vi "launcher.vi"(5 "RPM Control":dbl(knob) scale=0.0..3600.0, 6 "Stall":bool, 7 "Period (sec)":dbl) -> (0 "RPM":dbl(knob) scale=0.0..3000.0, 1 "RPM Steady?":bool, 3 "Motor Output":dbl(slide) scale=0.0..1.0)   [LabVIEW 2011]
uses:
  Robot Global Data.vi
  <vilib>/addons/control/pid/pid.llb/PID (DBL).vi
  <vilib>/addons/control/pid/NI_PID_pid.lvlib
panel:
  out "RPM Tolerance":dbl=25.0
  in  "PID Floor":dbl(knob)=609.2841617797657 scale=0.0..1000.0
  out "RPM High":bool
  out "RPM Low":bool
  out "1 RPM":bool
  out "5 RPM":bool
  out "2 RPM":bool
  out "8 RPM":bool
  out "7 RPM":bool
  out "6 RPM":bool
  out "4 RPM":bool
  out "3 RPM":bool
  out "RPM Control Response":cluster{"RPM Control 2":dbl, dbl, dbl}(graph)
  in  "Prop (like D)":dbl(knob)=0.002835162167809198 scale=0.0..0.01
  in  "Int (like P)":dbl(knob)=0.013165882226819458 scale=0.0..0.2
  in  "Deriv (not used)":dbl(knob) scale=0.0..0.01
  out "PID Output":dbl(graph)
  # "CIM: P=0.00192, I=0.00933, D=0.0"
  # "BB775: P=0.00283, I=0.01312, D=0.0"
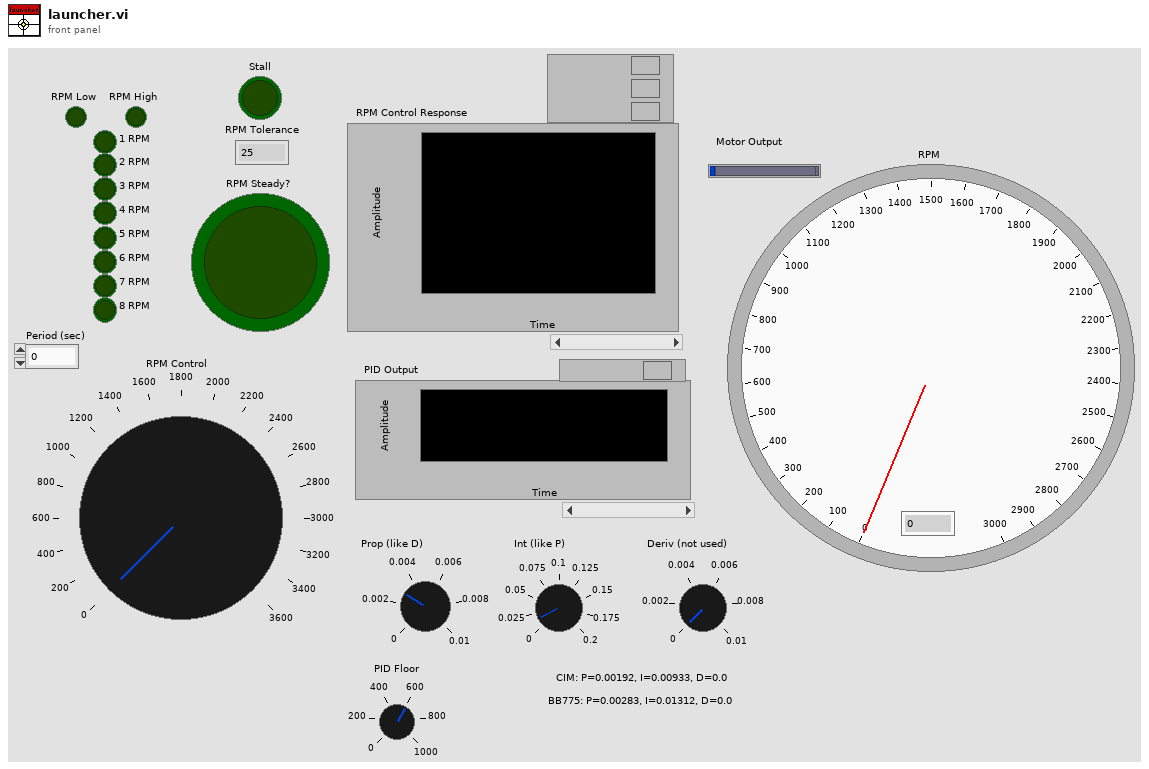
[diagram p1: front panel]
types:
  T1 = cluster{"Prop (like D)":dbl, "Int (like P)":dbl, "Deriv (not used)":dbl}
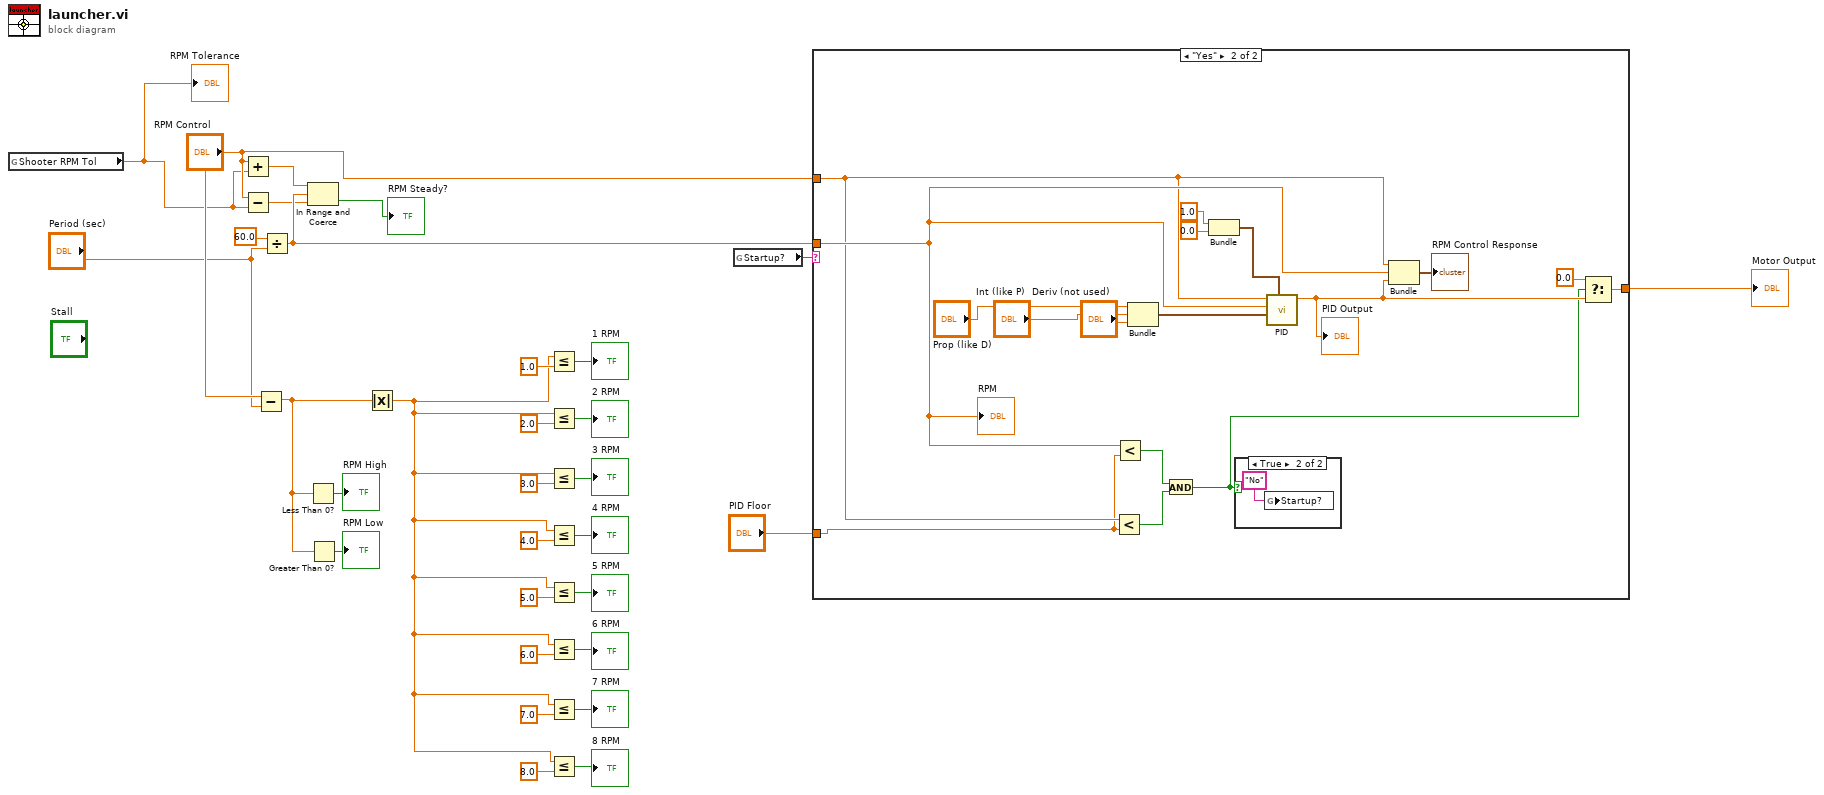
[diagram p0: block diagram]
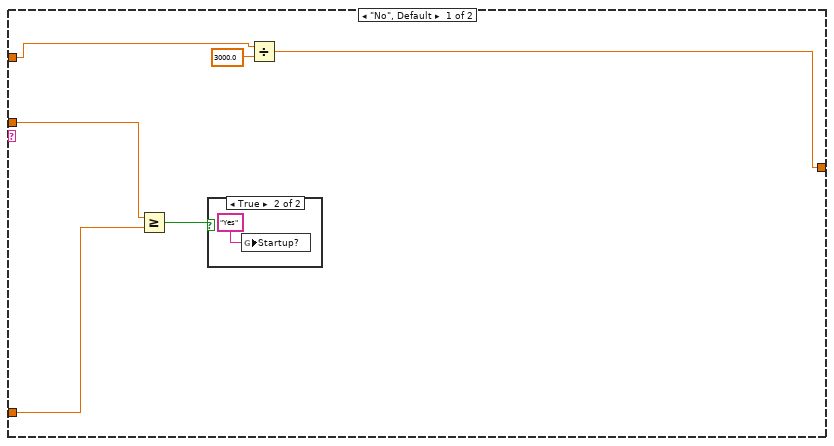
[diagram p2: hidden frame]
diagram:
  n1 = global read "Robot Global Data.vi" "Shooter RPM Tol"() -> (w1:dbl)
  "RPM Tolerance" <- w1
  n2 = Add(x="RPM Control", y=w1) -> (x+y=w26:dbl)
  n3 = Subtract(x="RPM Control", y=w1) -> (x-y=w27:dbl)
  n4 = Subtract(x="RPM Control", y="Period (sec)") -> (x-y=w6:dbl)
  n5 = Divide(x=60.0 ("y"), y="Period (sec)") -> (x/y=w29:dbl)
  n6 = In Range and Coerce(upper limit=w26, x=w29, lower limit=w27) -> (In Range?=→"RPM Steady?":bool)  [unwired: 1 out]
  n7 = Less Than 0?(x=w6) -> (x < 0?=→"RPM High":bool)
  n8 = Greater Than 0?(x=w6) -> (x > 0?=→"RPM Low":bool)
  n9 = Absolute Value(x=w6) -> (abs(x)=w9:dbl)
  n10 = Less Or Equal?(x=w9, y=1.0) -> (x <= y?=→"1 RPM":bool)
  n11 = Less Or Equal?(x=w9, y=2.0) -> (x <= y?=→"2 RPM":bool)
  n12 = Less Or Equal?(x=w9, y=3.0) -> (x <= y?=→"3 RPM":bool)
  n13 = Less Or Equal?(x=w9, y=4.0) -> (x <= y?=→"4 RPM":bool)
  n14 = Less Or Equal?(x=w9, y=5.0) -> (x <= y?=→"5 RPM":bool)
  n15 = Less Or Equal?(x=w9, y=6.0) -> (x <= y?=→"6 RPM":bool)
  n16 = Less Or Equal?(x=w9, y=7.0) -> (x <= y?=→"7 RPM":bool)
  n17 = Less Or Equal?(x=w9, y=8.0) -> (x <= y?=→"8 RPM":bool)
  n18 = global read "Robot Global Data.vi" "Startup?"() -> (w30:string)
  n19 = case shown="\"Yes\"" w30 {
    tunnel: [w37 w55] -> w3
    tunnel: w29 -> [w32 w42]
    tunnel: "RPM Control" -> [w36 w41]
    tunnel: "PID Floor" -> [w33 w40]
    frame "No", Default {
      n20 = Greater Or Equal?(x=w32, y=w33) -> (x >= y?=w34:bool)
      n21 = case shown="True" w34 {
        frame False {
        }
        frame True {
          n22 = global write "Robot Global Data.vi" "Startup?"("Yes" ("Startup?")) -> ()
        }
      }
      n23 = Divide(x=w36, y=3000.0) -> (x/y=w37:dbl)
    }
    frame "Yes" {
      n24 = Less?(x=w41, y=w40) -> (x < y?=w43:bool)
      n25 = Less?(x=w42, y=w40) -> (x < y?=w44:bool)
      n26 = Bundle("Prop (like D)"="Prop (like D)", "Int (like P)"="Int (like P)", "Deriv (not used)"="Deriv (not used)") -> (w49:T1)  [unwired: 1 out]
      n27 = And(x=w44, y=w43) -> (x .and. y?=w39:bool)
      n28 = Bundle("x"=1.0, 0.0) -> (w46:cluster{"x":dbl, dbl})  [unwired: 1 out]
      n29 = case shown="True" w39 {
        frame False {
        }
        frame True {
          n30 = global write "Robot Global Data.vi" "Startup?"("No" ("Startup?")) -> ()
        }
      }
      n31 = call-poly <vilib>:"PID.vi"("output range"=w46, "PID gains"=w49, "process variable"=w42, "setpoint"=w41) -> ("output"=w45:dbl)  [unwired: 2 in, 5 out]
      "PID Output" <- w45
      n32 = Bundle("RPM Control"=w41, w42, "output"=w45) -> (→"RPM Control Response":cluster{"RPM Control":dbl, dbl, "output":dbl})  [unwired: 1 out]
      n33 = Select(t=0.0, s=w39, f=w45) -> (s? t:f=w55:dbl)
      "RPM" <- w42
    }
  }
  "Motor Output" <- w3
